vi "Vision ProcessingCheeto.vi"(4 "error in (no error)":errorcluster, 7 "Image Size Gear":T2=enum."160x120") -> ()   [LabVIEW 2016]
doc: "This VI runs in parallel to other tasks. It gets images from the camera, processes them for color or shape and use that information to affect robot behavior."
uses:
  Vision Support VIs/Camera Types.ctl
  <vilib>/Rock Robotics/WPI/Camera/WPI_CameraImageSize.ctl
  <vilib>/vision/Measure.llb/Edge Options.ctl
  <vilib>/vision/Measure.llb/Edge Polarity.ctl
  <vilib>/Rock Robotics/WPI/Camera/WPI_CameraWhite Balance Values.ctl
  <vilib>/Rock Robotics/WPI/Camera/WPI_CameraExposure Values.ctl
  <vilib>/Rock Robotics/WPI/Camera/WPI_CameraFrameRate.ctl
  <vilib>/Platform/TimedLoop/XDataNode/timing_clust.ctl
  <vilib>/Platform/TimedLoop/XDataNode/nitl_modes.ctl
  <vilib>/Platform/TimedLoop/XDataNode/wakeup.ctl
  Robot Global Data.vi
  <vilib>/platform/TimedLoop/XDataNode/XDataNode.xnode
  <vilib>/vision/NI_Vision_Development_Module.lvlib
  <vilib>/Platform/TimedLoop/XDataNode/XDNodeRunTimeDep.lvlib
panel:
  out "Distance (lateral) 2":dbl
  out "Distance (lateral) 1":dbl
  out "Gear Sorted Data":dbl[][](array[numeric])
  out "Original Image 3":T1(plugin-control)
  in  "error in (no error) 3":errorcluster
  in  "Image Size 2":T2=enum."320x240"
  in  "Image Size":T2=enum."320x240"
  in  "error in (no error) 2":errorcluster
  out "Original Image 2":T1(plugin-control)
  out "Gear Yaw Delta":dbl=-5.600000000000001
  in  "Boiler boresight":dbl=8.65
  in  "Edge Options Gear":T3={"Edge Polarity"=0, "Kernel Size"=3, "Width"=3, "Minimum Edge Strength"=15.0, "Interpolation Type"=enum."Bilinear Fixed", "Data Processing Method"=enum."Average"} {"Edge Polarity" items=["All Edges", "Rising Edges", "Falling Edges"]; "Minimum Edge Strength" format="%.2f"; "Width" step=2; "Kernel Size" step=2}
  in  "Gear boresight":dbl=24.9
  in  "Factor to Distance":dbl=12.0
  in  "Ball?":bool=TRUE
  in  "LED Color Ball":T5={"Hue"={190.47824477034428, 247.1686130718606}, "Sat"={57.67857142857144, 203.39285714285714}, "Val"={27.32142857142858, 255.0}} {"Hue" scale=0.0..255.0 scale format="%#_3g"}
  in  "Brightness":i32=30
  in  "Exposure (%)":dbl format="%#_13g"
  in  "Color Temp (K)":dbl=4000.0 format="%#_13g"
  in  "Edge Options":T3={"Edge Polarity"=0, "Kernel Size"=3, "Width"=3, "Minimum Edge Strength"=2.0, "Interpolation Type"=enum."Bilinear Fixed", "Data Processing Method"=enum."Average"} {"Edge Polarity" items=["All Edges", "Rising Edges", "Falling Edges"]; "Minimum Edge Strength" format="%.2f"; "Width" step=2; "Kernel Size" step=2}
  in  "Size Limit %":dbl=0.04 format="%#_13g"
  in  "Cal Turret":bool
  out "Calibration error 2":errorcluster={"status"=TRUE, "code"=-1074396074, "source"=""}
  out "Physical Paths":string[](array[string])=["-0_1_1_1_0", "-0_1_2_1_0"]
  out "Logical Paths":string[](array[string])=["video0", "video1"]
  out "Gear Valid":bool
  out "Boiler Yaw Delta":dbl=-8.499999999999998
  out "Boiler Valid":bool
  out "Boiler Distance":dbl=inf
  in  "Angle":enum16{"Horizontal", "Vertical", "Diagonal"}(ring)=enum."Vertical"
  in  "Gear?":bool
  in  "Image SizeTurr":T2=enum."160x120"
  in  "Score Cutoff Turret":dbl=70.0
  out "Gear Distance":dbl=inf
  in  "FOV":cluster{"X (degrees)":dbl, "Y (degrees)":dbl}={"X (degrees)"=34.3, "Y (degrees)"=61.0}
  in  "Height":T6={"Hc (GND to lense)"=12.5, "Ht (GND to CTR)"=0.0}
  in  "LED Color Target":T5={"Hue"={217.1650671807445, 7.296259223023774}, "Sat"={115.35714285714286, 255.0}, "Val"={21.25000000000001, 255.0}} {"Hue" scale=0.0..255.0 scale format="%#_3g"}
  in  "Camera Type":T7=enum."1013"
  in  "Score Cutoff %":dbl=50.0
  in  "Particles":dbl=5.0
  in  "Color Mode":u16(ring)=3 items=["RGB", "HSL", "HSV", "HSI"]
  in  "Use Calibration":bool
  out "Calibration error":errorcluster
  in  "Line Border":cluster{"Top":dbl, "Bottom":dbl}={"Top"=6.0, "Bottom"=1.0}
  in  "Display Original":bool=TRUE
  in  "Display Mask":bool=TRUE
  out "Mask":T1(plugin-control)
  out "Original Image":T1(plugin-control)
  out "loop ms":u32=200
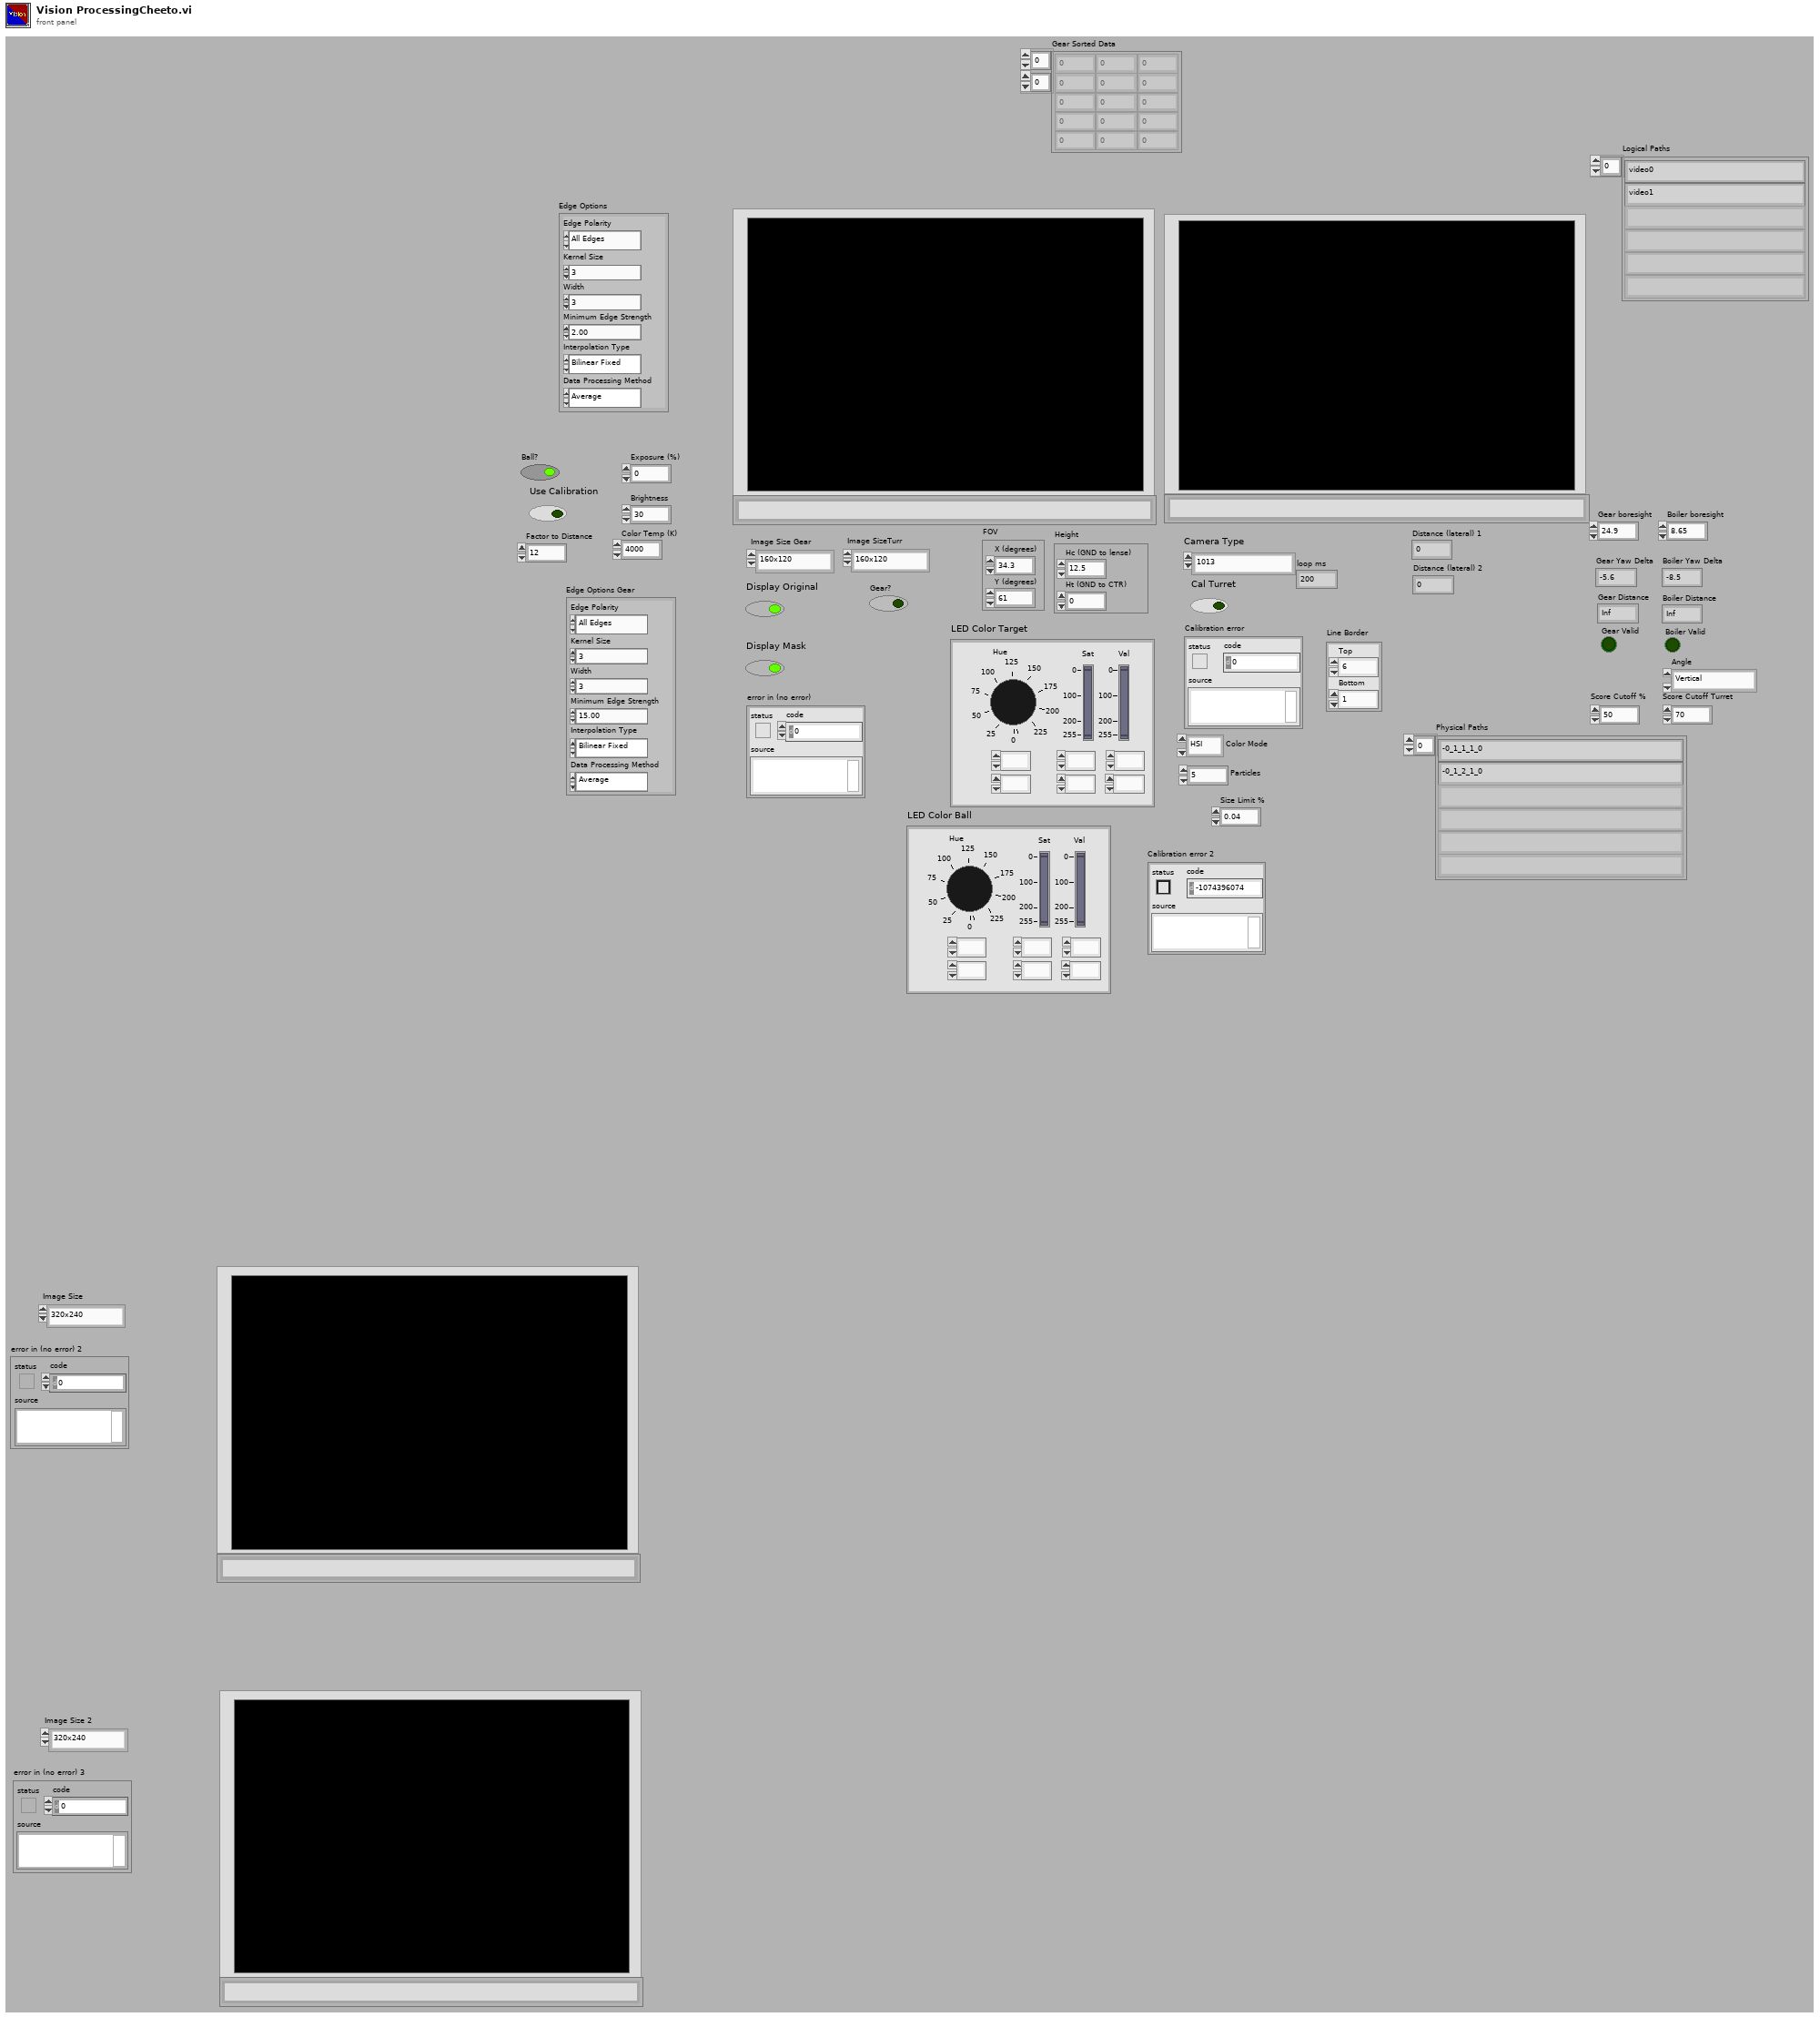
[diagram p1: front panel]
types:
  T1 = typedef "IMAQ Image.ctl" = refnum<image>
  T2 = typedef "WPI_CameraImageSize.ctl" = enum16{"640x480", "320x240", "160x120", "Custom"}
  T3 = typedef "Edge Options.ctl" = cluster{"Edge Polarity":T4, "Kernel Size":u32, "Width":u32, "Minimum Edge Strength":sgl, "Interpolation Type":enum32{"Zero Order", "Bilinear", "Quadratic", "Cubic", "Bilinear Fixed"}, "Data Processing Method":enum32{"Average", "Median"}}
  T4 = typedef "Edge Polarity.ctl" = u32
  T5 = cluster{"Hue":cluster{dbl, dbl}, "Sat":cluster{dbl, dbl}, "Val":cluster{dbl, dbl}}
  T6 = cluster{"Hc (GND to lense)":dbl, "Ht (GND to CTR)":dbl}
  T7 = typedef "Camera Types.ctl" = enum16{"206", "1011", "1013", "MS HD3000 square", "MS HD3000 640x480"}
  T8 = typedef "WPI_CameraFrameRate.ctl" = u32
  T9 = typedef "WPI_CameraExposure Values.ctl" = enum16{"Auto", "Flicker-free 50 Hz", "Flicker-free 60 Hz", "Hold current", "Custom"}
  T10 = typedef "WPI_CameraWhite Balance Values.ctl" = enum16{"Auto", "Fixed indoor", "Fixed outdoor 1", "Fixed outdoor 2", "Fixed fluorescent 1", "Fixed fluorescent 2", "Hold current", "Custom"}
  T11 = typedef "XDNodeRunTimeDep.lvlib/timing_clust.ctl" = cluster{"Expected End [f-1]":u64, "Actual End [f-1]":u64, "Finished Late? [f-1]":bool, "Expected End [i-1]":u64, "Actual End [i-1]":u64, "Finished Late? [i-1]":bool, "Expected Start [i]":u64, "Actual Start [i]":u64, "Expected Start [f]":u64, "Actual Start [f]":u64, "Source Name":string, "Structure Name":string, "Period":i64, "Deadline":i64, "Offset":i64, "Start":i64, "Priority":i32, "Timeout":i32, "Mode":T12, "Wakeup Reason":T13, "Error":errorcluster, "Source Type":string, "Secondary Source Type":string, "Global End Time":u64, "Global Start Time":u64, "Frame Duration":u64, "Iteration Duration":u64, "Assigned CPU":i32, "I/O Scan Engine Mode":u32}
  T12 = typedef "XDNodeRunTimeDep.lvlib/nitl_modes.ctl" = enum32{"No Change", "Process missed periods, maintain original phase", "Discard missed periods, maintain original phase", "Process missed periods, ignore original phase", "Discard missed periods, ignore original phase"}
  T13 = typedef "XDNodeRunTimeDep.lvlib/wakeup.ctl" = enum32{"Normal", "Aborted", "Asynchronous wakeup", "Timing source error", "Timed loop error", "Timeout"}
  T14 = typedef "Image Type" = u32
  T15 = typedef "WPI_CameraDevRef.ctl" = cluster{"Camera Address":string, "CameraStatus":errorcluster}
  T16 = typedef "Particle Parameters" = i32
  T17 = cluster{"Left":dbl, "Top":dbl, "Right":dbl, "Bottom":dbl}
  T18 = cluster{"Distance (ft)":dbl, "Score":dbl, "Normalized":cluster{"Center":cluster{dbl, dbl}, "Rectangle":cluster{"Numeric":dbl, "Numeric 2":dbl, "Numeric 3":dbl, "Numeric 5":dbl}}, "Pixels":cluster{"Center":cluster{dbl, dbl}, "Rectangle":cluster{"Numeric":dbl, "Numeric 2":dbl, "Numeric 3":dbl, "Numeric 5":dbl}}}
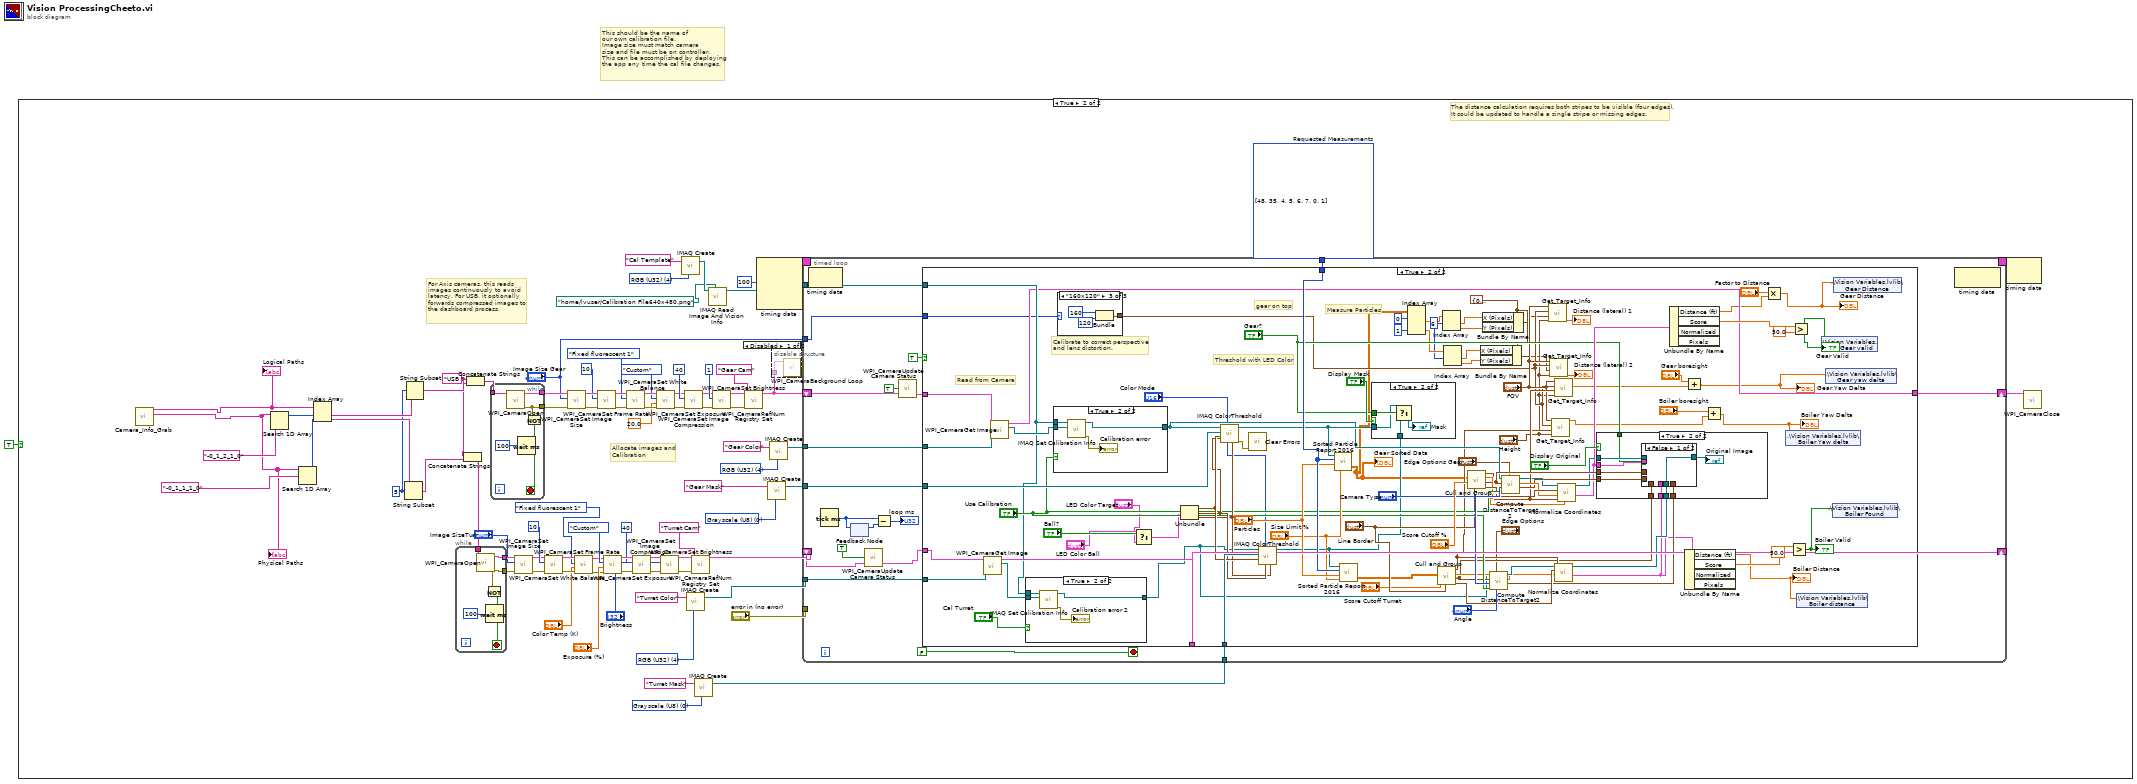
[diagram p0: block diagram]
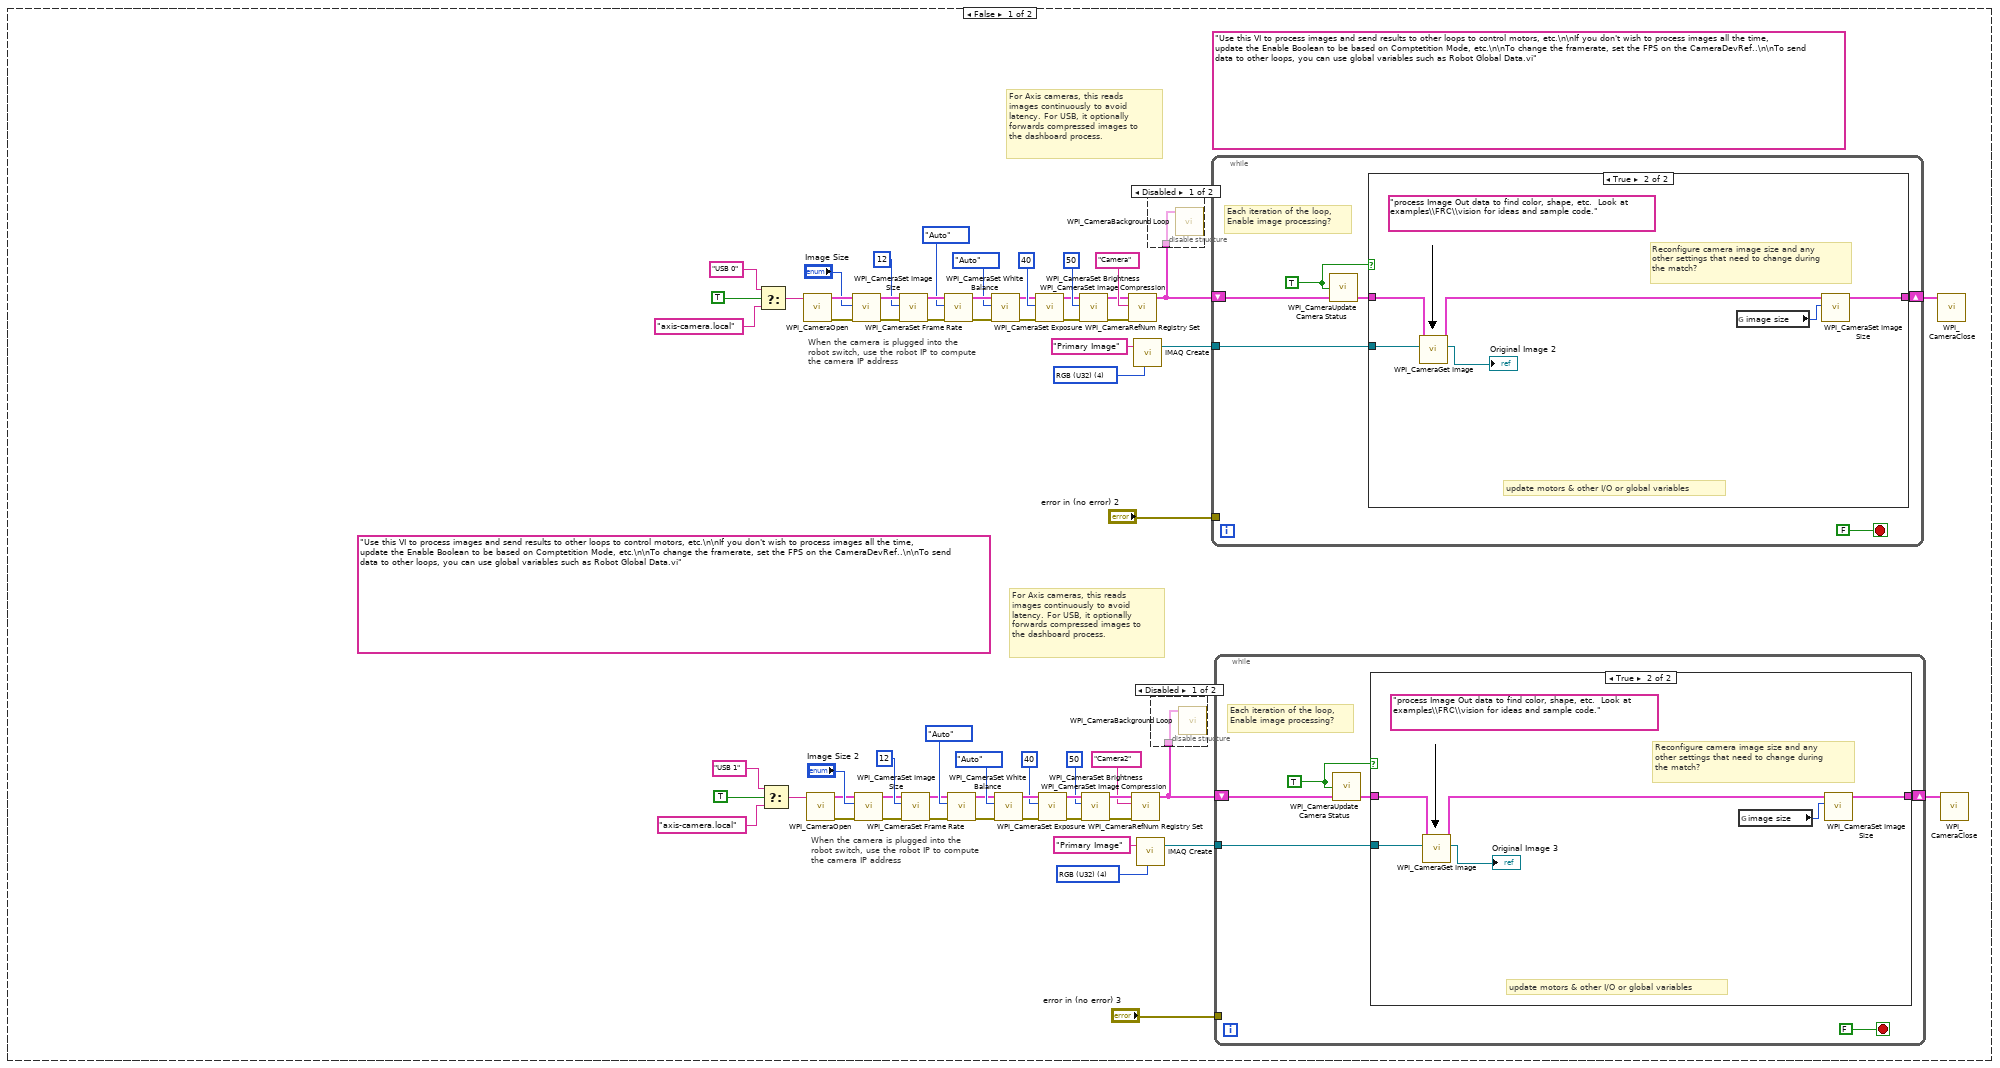
[diagram p2: hidden frame]
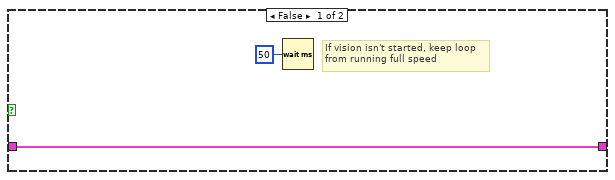
[diagram p4: hidden frame]
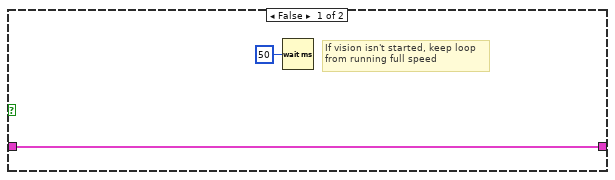
[diagram p6: hidden frame]
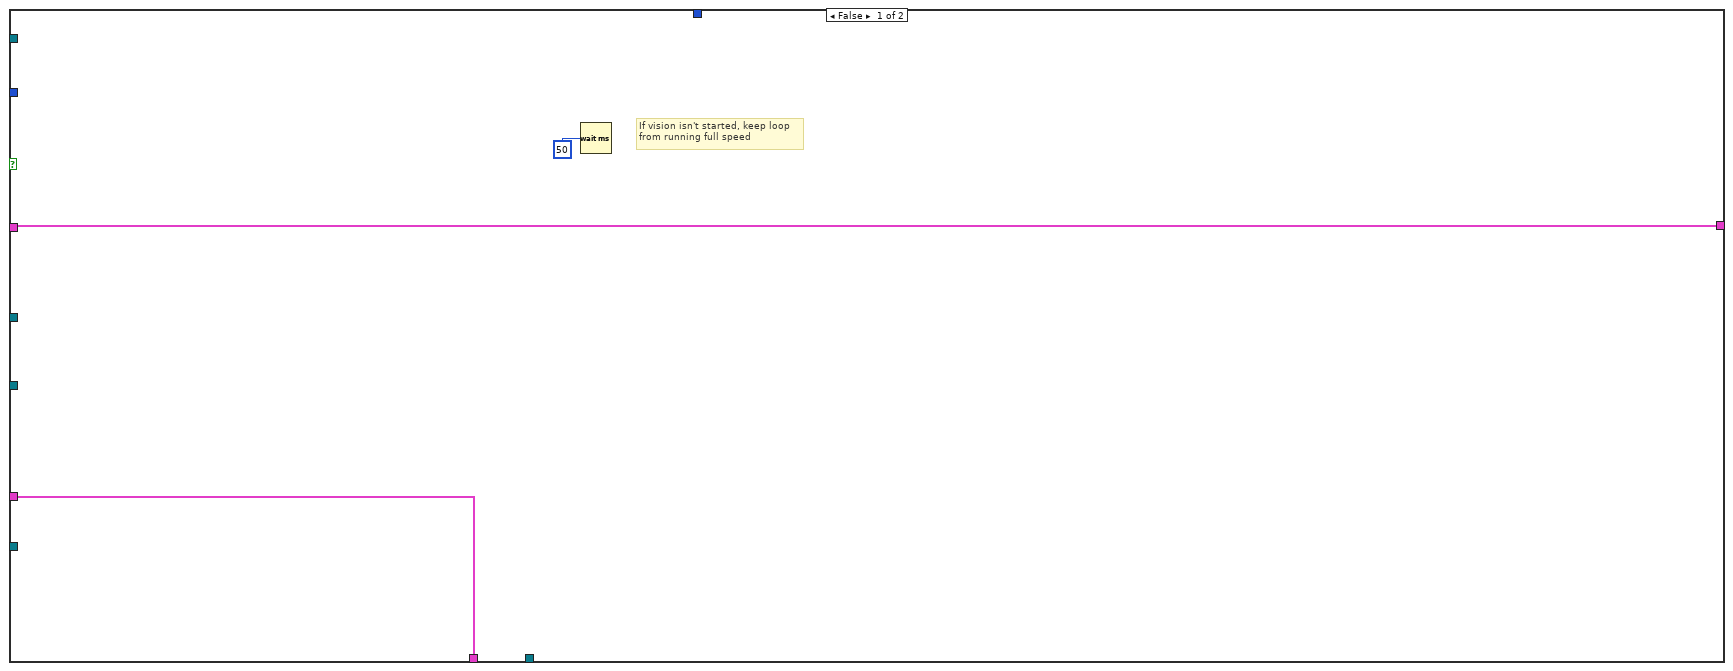
[diagram p7: hidden frame]
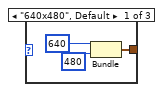
[diagram p8: hidden frame]
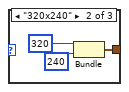
[diagram p9: hidden frame]
diagram:
  # "This should be the name of \nour own calibration file.\nImage size must match camera\nsize and file must be on controller.\nThis can be accomplished by deploying\nthe app any time the cal file changes."
  n1 = case shown="True" TRUE {
    frame False {
      (unwired) "Use this VI to process images and send results to other loops to control motors, etc.\n\nIf you don't wish to process images all the time, update the Enable Boolean to be based on Comptetition Mode, etc.\n\nTo change the framerate, set the FPS on the CameraDevRef..\n\nTo send data to other loops, you can use global variables such as Robot Global Data.vi"
      w2 = T14 4 items=["Grayscale (U8)", "Grayscale (I16)", "Grayscale (SGL)", "Complex (CSG)", "RGB (U32)", "HSL (U32)", "RGB (U64)"] ("Image Type")
      (unwired) "Use this VI to process images and send results to other loops to control motors, etc.\n\nIf you don't wish to process images all the time, update the Enable Boolean to be based on Comptetition Mode, etc.\n\nTo change the framerate, set the FPS on the CameraDevRef..\n\nTo send data to other loops, you can use global variables such as Robot Global Data.vi"
      w63 = T14 4 items=["Grayscale (U8)", "Grayscale (I16)", "Grayscale (SGL)", "Complex (CSG)", "RGB (U32)", "HSL (U32)", "RGB (U64)"] ("Image Type")
      # "When the camera is plugged into the\nrobot switch, use the robot IP to compute\nthe camera IP address"
      # "For Axis cameras, this reads\nimages continuously to avoid\nlatency. For USB, it optionally\nforwards compressed images to\nthe dashboard process."
      # "When the camera is plugged into the\nrobot switch, use the robot IP to compute\nthe camera IP address"
      # "For Axis cameras, this reads\nimages continuously to avoid\nlatency. For USB, it optionally\nforwards compressed images to\nthe dashboard process."
      n2 = Select(t="USB 0" ("format string"), s=TRUE ("dot notation? (F)"), f="axis-camera.local" ("format string")) -> (s? t:f=w34:string)
      n3 = Select(t="USB 1" ("format string"), s=TRUE ("dot notation? (F)"), f="axis-camera.local" ("format string")) -> (s? t:f=w31:string)
      n4 = call <vilib>:"WPI_CameraOpen.vi"("Camera Address"=w34) -> ("error out"=w51:errorcluster, "CameraDevRef"=w52:T15)  [unwired: 1 in, 8 out]
      n5 = call <vilib>:"WPI_CameraOpen.vi"("Camera Address"=w31) -> ("error out"=w14:errorcluster, "CameraDevRef"=w13:T15)  [unwired: 1 in, 8 out]
      n6 = call <vilib>:"WPI_CameraSet Image Size.vi"("error in (no error)"=w51, "Image Size"="Image Size", "CameraDevRef"=w52) -> ("error out"=w50:errorcluster, "CameraDevRef Out"=w53:T15)  [unwired: 1 in, 6 out]
      n7 = call <vilib>:"WPI_CameraSet Image Size.vi"("error in (no error)"=w14, "Image Size"="Image Size 2", "CameraDevRef"=w13) -> ("error out"=w15:errorcluster, "CameraDevRef Out"=w12:T15)  [unwired: 1 in, 6 out]
      n8 = call <vilib>:"WPI_CameraSet Frame Rate.vi"("error in (no error)"=w50, "Frame Rate (fps)"=T8 12, "CameraDevRef"=w53) -> ("error out"=w49:errorcluster, "CameraDevRef Out"=w55:T15)  [unwired: 7 out]
      n9 = call <vilib>:"WPI_CameraSet Frame Rate.vi"("error in (no error)"=w15, "Frame Rate (fps)"=T8 12, "CameraDevRef"=w12) -> ("error out"=w16:errorcluster, "CameraDevRef Out"=w10:T15)  [unwired: 7 out]
      n10 = call <vilib>:"WPI_CameraSet White Balance.vi"("error in (no error)"=w49, "White Balance"=WPI_CameraWhite_Balance_Values."Auto", "CameraDevRef"=w55) -> ("error out"=w48:errorcluster, "CameraDevRef Out"=w54:T15)  [unwired: 1 in, 6 out]
      n11 = call <vilib>:"WPI_CameraSet White Balance.vi"("error in (no error)"=w16, "White Balance"=WPI_CameraWhite_Balance_Values."Auto", "CameraDevRef"=w10) -> ("error out"=w17:errorcluster, "CameraDevRef Out"=w11:T15)  [unwired: 1 in, 6 out]
      n12 = call <vilib>:"WPI_CameraSet Exposure.vi"("error in (no error)"=w48, "Exposure"=WPI_CameraExposure_Values."Auto", "CameraDevRef"=w54) -> ("error out"=w47:errorcluster, "CameraDevRef Out"=w57:T15)  [unwired: 1 in, 6 out]
      n13 = call <vilib>:"WPI_CameraSet Exposure.vi"("error in (no error)"=w17, "Exposure"=WPI_CameraExposure_Values."Auto", "CameraDevRef"=w11) -> ("error out"=w18:errorcluster, "CameraDevRef Out"=w8:T15)  [unwired: 1 in, 6 out]
      n14 = call <vilib>:"WPI_CameraSet Image Compression.vi"("error in (no error)"=w47, "Compression"=40, "CameraDevRef"=w57) -> ("error out"=w46:errorcluster, "CameraDevRef Out"=w56:T15)  [unwired: 7 out]
      n15 = call <vilib>:"WPI_CameraSet Image Compression.vi"("error in (no error)"=w18, "Compression"=40, "CameraDevRef"=w8) -> ("error out"=w19:errorcluster, "CameraDevRef Out"=w9:T15)  [unwired: 7 out]
      n16 = call <vilib>:"WPI_CameraSet Brightness.vi"("error in (no error)"=w46, "Brightness"=50, "CameraDevRef"=w56) -> ("error out"=w44:errorcluster, "CameraDevRef Out"=w45:T15)  [unwired: 7 out]
      n17 = call <vilib>:"WPI_CameraSet Brightness.vi"("error in (no error)"=w19, "Brightness"=50, "CameraDevRef"=w9) -> ("error out"=w21:errorcluster, "CameraDevRef Out"=w20:T15)  [unwired: 7 out]
      n18 = call <vilib>:"WPI_CameraRefNum Registry Set.vi"("error in (no error)"=w44, "refnum name"="Camera", "CameraDevRef"=w45) -> ("CameraDevRef"=w40:T15)  [unwired: 1 in, 7 out]
      n19 = call <vilib>:"WPI_CameraRefNum Registry Set.vi"("error in (no error)"=w21, "refnum name"="Camera2", "CameraDevRef"=w20) -> ("CameraDevRef"=w25:T15)  [unwired: 1 in, 7 out]
      n20 = call "IMAQ Create"("Image Name"="Primary Image", "Image Type"=w63) -> ("New Image"=w61:T1)  [unwired: 2 in, 2 out]
      n21 = call "IMAQ Create"("Image Name"="Primary Image", "Image Type"=w2) -> ("New Image"=w4:T1)  [unwired: 2 in, 2 out]
      n22 = disable-structure shown="Disabled" {
        disable-tunnel: w40 -> [w79 _]
        frame Disabled {
          n23 = call <vilib>:"WPI_CameraBackground Loop.vi"("CameraDevRef"=w79) -> ()  [unwired: 11 in]
        }
        frame Enabled {
        }
      }
      n24 = disable-structure shown="Disabled" {
        disable-tunnel: w25 -> [w64 _]
        frame Disabled {
          n25 = call <vilib>:"WPI_CameraBackground Loop.vi"("CameraDevRef"=w64) -> ()  [unwired: 11 in]
        }
        frame Enabled {
        }
      }
      n26 = while {
        shift-right: [w84] -> w38
        shift-left: w40 -> [w82]
        tunnel: w61 -> [w83]
        tunnel: "error in (no error) 2" -> [_]
        stop <- FALSE stop-if-true
        w80 = TRUE
        # "Each iteration of the loop,\nEnable image processing?"
        n27 = call <vilib>:"WPI_CameraUpdate Camera Status.vi"("CameraDevRef In"=w82, "Enable Vision"=w80) -> ("CameraDevRef Out"=w81:T15)  [unwired: 3 in]
        n28 = case shown="True" w80 {
          tunnel: w83 -> [_ w92]
          tunnel: [w87 w93] -> w84
          tunnel: w81 -> [w87 w90]
          frame False {
            # "If vision isn't started, keep loop\nfrom running full speed"
            n29 = Wait (ms)(milliseconds to wait=u32 50) -> ()  [unwired: 1 out]
          }
          frame True {
            (unwired) "process Image Out data to find color, shape, etc.  Look at examples\\FRC\\vision for ideas and sample code."
            # "update motors & other I/O or global variables"
            # "Reconfigure camera image size and any\nother settings that need to change during\nthe match?"
            n30 = call <vilib>:"WPI_CameraGet Image.vi"("Image"=w92, "CameraDevRef"=w90) -> ("Image Out"=→"Original Image 2":T1, "CameraDevRef Out"=w89:T15)  [unwired: 1 in, 7 out]
            n31 = global read "Robot Global Data.vi" "image size"() -> (w91:T2)
            n32 = call <vilib>:"WPI_CameraSet Image Size.vi"("Image Size"=w91, "CameraDevRef"=w89) -> ("CameraDevRef Out"=w93:T15)  [unwired: 2 in, 7 out]
          }
        }
      }
      n33 = while {
        shift-right: [w69] -> w27
        shift-left: w25 -> [w67]
        tunnel: w4 -> [w68]
        tunnel: "error in (no error) 3" -> [_]
        stop <- FALSE stop-if-true
        w65 = TRUE
        # "Each iteration of the loop,\nEnable image processing?"
        n34 = call <vilib>:"WPI_CameraUpdate Camera Status.vi"("CameraDevRef In"=w67, "Enable Vision"=w65) -> ("CameraDevRef Out"=w66:T15)  [unwired: 3 in]
        n35 = case shown="True" w65 {
          tunnel: w68 -> [_ w77]
          tunnel: [w72 w78] -> w69
          tunnel: w66 -> [w72 w75]
          frame False {
            # "If vision isn't started, keep loop\nfrom running full speed"
            n36 = Wait (ms)(milliseconds to wait=u32 50) -> ()  [unwired: 1 out]
          }
          frame True {
            (unwired) "process Image Out data to find color, shape, etc.  Look at examples\\FRC\\vision for ideas and sample code."
            # "update motors & other I/O or global variables"
            # "Reconfigure camera image size and any\nother settings that need to change during\nthe match?"
            n37 = call <vilib>:"WPI_CameraGet Image.vi"("Image"=w77, "CameraDevRef"=w75) -> ("Image Out"=→"Original Image 3":T1, "CameraDevRef Out"=w74:T15)  [unwired: 1 in, 7 out]
            n38 = global read "Robot Global Data.vi" "image size"() -> (w76:T2)
            n39 = call <vilib>:"WPI_CameraSet Image Size.vi"("Image Size"=w76, "CameraDevRef"=w74) -> ("CameraDevRef Out"=w78:T15)  [unwired: 2 in, 7 out]
          }
        }
      }
      n40 = call <vilib>:"WPI_CameraClose.vi"("CameraDevRef"=w38) -> ()  [unwired: 1 in, 10 out]
      n41 = call <vilib>:"WPI_CameraClose.vi"("CameraDevRef"=w27) -> ()  [unwired: 1 in, 10 out]
    }
    frame True {
      w108 = "USB " ("string")
      w110 = 5 ("offset (0)")
      w118 = T14 0 items=["Grayscale (U8)", "Grayscale (I16)", "Grayscale (SGL)", "Complex (CSG)", "RGB (U32)", "HSL (U32)", "RGB (U64)", "Grayscale (U16)"] ("Image Type")
      w120 = T14 4 items=["Grayscale (U8)", "Grayscale (I16)", "Grayscale (SGL)", "Complex (CSG)", "RGB (U32)", "HSL (U32)", "RGB (U64)", "Grayscale (U16)"] ("Image Type")
      w168 = T14 4 items=["Grayscale (U8)", "Grayscale (I16)", "Grayscale (SGL)", "Complex (CSG)", "RGB (U32)", "HSL (U32)", "RGB (U64)", "Grayscale (U16)"] ("Image Type")
      w173 = T14 0 items=["Grayscale (U8)", "Grayscale (I16)", "Grayscale (SGL)", "Complex (CSG)", "RGB (U32)", "HSL (U32)", "RGB (U64)", "Grayscale (U16)"] ("Image Type")
      w174 = T14 4 items=["Grayscale (U8)", "Grayscale (I16)", "Grayscale (SGL)", "Complex (CSG)", "RGB (U32)", "HSL (U32)", "RGB (U64)", "Grayscale (U16)"] ("Image Type")
      w170 = T16[] [48, 35, 4, 5, 6, 7, 0, 1] items=["Center of Mass X", "Center of Mass Y", "First Pixel X", "First Pixel Y", "Bounding Rect Left", "Bounding Rect Top", "Bounding Rect Right", "Bounding Rect Bottom", "Max Feret Diameter Start X", "Max Feret Diameter Start Y", "Max Feret Diameter End X", "Max Feret Diameter End Y", "Max Horiz. Segment Length Left", "Max Horiz. Segment Length Right", "Max Horiz. Segment Length Row", "-", "Bounding Rect Width", "Bounding Rect Height", "Bounding Rect Diagonal", "Perimeter", "Convex Hull Perimeter", "Holes' Perimeter", "Max Feret Diameter", "Equivalent Ellipse Major Axis", "Equivalent Ellipse Minor Axis", "Equivalent Ellipse Minor Axis (Feret)", "Equivalent Rect Long Side", "Equivalent Rect Short Side", "Equivalent Rect Diagonal", "Equivalent Rect Short Side (Feret)", "Average Horiz. Segment Length", "Average Vert. Segment Length", "Hydraulic Radius", "Waddel Disk Diameter", "-", "Area", "Holes' Area", "Particle & Holes' Area", "Convex Hull Area", "Image Area", "-", "Number of Holes", "Number of Horiz. Segments", "Number of Vert. Segments", "-", "Orientation", "Max Feret Diameter Orientation", "-", "% Area/Image Area", "% Area/(Particle & Holes' Area)", "Ratio of Equivalent Ellipse Axes", "Ratio of Equivalent Rect Sides", "-", "Elongation Factor", "Compactness Factor", "Heywood Circularity Factor", "Type Factor", "-", "Sum X", "Sum Y", "Sum XX", "Sum XY", "Sum YY", "Sum XXX", "Sum XXY", "Sum XYY", "Sum YYY", "-", "Moment of Inertia XX", "Moment of Inertia XY", "Moment of Inertia YY", "Moment of Inertia XXX", "Moment of Inertia XXY", "Moment of Inertia XYY", "Moment of Inertia YYY", "Norm. Moment of Inertia XX", "Norm. Moment of Inertia XY", "Norm. Moment of Inertia YY", "Norm. Moment of Inertia XXX", "Norm. Moment of Inertia XXY", "Norm. Moment of Inertia XYY", "Norm. Moment of Inertia YYY", "Hu Moment 1", "Hu Moment 2", "Hu Moment 3", "Hu Moment 4", "Hu Moment 5", "Hu Moment 6", "Hu Moment 7"]  # Requested Measurements
      # "For Axis cameras, this reads\nimages continuously to avoid\nlatency. For USB, it optionally\nforwards compressed images to\nthe dashboard process."
      # "Allocate images and\nCalibration"
      # "The distance calculation requires both stripes to be visible (four edges).\nIt could be updated to handle a single stripe or missing edges."
      n42 = call <userlib>:"Camera_Info_Grab.vi"() -> ("Physical Paths"=w102:string[], "Logical Paths"=w103:string[])  [unwired: 10 in]
      "Logical Paths" <- w103
      "Physical Paths" <- w102
      n43 = Search 1D Array(1D array=w102, element="-0_1_2_1_0") -> (index of element=w114:i32)  [unwired: 1 in]
      n44 = Search 1D Array(1D array=w102, element="-0_1_1_1_0") -> (index of element=w113:i32)  [unwired: 1 in]
      n45 = Index Array(array=w103, index #1=w114, index #2=w113) -> (element #1=w112:string, element #2=w111:string)
      n46 = String Subset(string=w111, offset (0)=w110) -> (substring=w107:string)  [unwired: 1 in]
      n47 = String Subset(string=w112, offset (0)=w110) -> (substring=w109:string)  [unwired: 1 in]
      n48 = Concatenate Strings(w108, w107) -> (w106:string)
      n49 = while {
        tunnel: [w341] -> w133
        tunnel: [w344] -> w132
        tunnel: w106 -> [w343]
        stop <- w340 stop-if-true
        n50 = call <vilib>:"WPI_CameraOpen.vi"("Camera Address"=w343) -> ("error out"=w341:errorcluster, "CameraDevRef"=w344:T15)  [unwired: 1 in, 8 out]
        n51 = Not(x=w341) -> (.not. x?=w340:bool)
        n52 = Wait (ms)(milliseconds to wait=u32 100) -> ()  [unwired: 1 out]
      }
      n53 = Concatenate Strings(w108, w109) -> (w105:string)
      n54 = while {
        tunnel: [w339] -> w155
        tunnel: [w336] -> w154
        tunnel: w105 -> [w338]
        stop <- w335 stop-if-true
        n55 = call <vilib>:"WPI_CameraOpen.vi"("Camera Address"=w338) -> ("error out"=w336:errorcluster, "CameraDevRef"=w339:T15)  [unwired: 1 in, 8 out]
        n56 = Wait (ms)(milliseconds to wait=u32 100) -> ()  [unwired: 1 out]
        n57 = Not(x=w336) -> (.not. x?=w335:bool)
      }
      n58 = call <vilib>:"WPI_CameraSet Image Size.vi"("error in (no error)"=w133, "Image Size"="Image SizeTurr", "CameraDevRef"=w132) -> ("error out"=w134:errorcluster, "CameraDevRef Out"=w131:T15)  [unwired: 1 in, 6 out]
      n59 = call <vilib>:"WPI_CameraSet Frame Rate.vi"("error in (no error)"=w134, "Frame Rate (fps)"=T8 10, "CameraDevRef"=w131) -> ("error out"=w98:errorcluster, "CameraDevRef Out"=w100:T15)  [unwired: 7 out]
      n60 = call <vilib>:"WPI_CameraSet Image Size.vi"("error in (no error)"=w154, "Image Size"="Image Size Gear", "CameraDevRef"=w155) -> ("error out"=w153:errorcluster, "CameraDevRef Out"=w156:T15)  [unwired: 1 in, 6 out]
      n61 = call <vilib>:"WPI_CameraSet White Balance.vi"("error in (no error)"=w98, "Color Temp (K)"="Color Temp (K)", "White Balance"=WPI_CameraWhite_Balance_Values."Fixed fluorescent 1", "CameraDevRef"=w100) -> ("error out"=w97:errorcluster, "CameraDevRef Out"=w99:T15)  [unwired: 6 in]
      n62 = call <vilib>:"WPI_CameraSet Frame Rate.vi"("error in (no error)"=w153, "Frame Rate (fps)"=T8 10, "CameraDevRef"=w156) -> ("error out"=w152:errorcluster, "CameraDevRef Out"=w158:T15)  [unwired: 7 out]
      n63 = call <vilib>:"WPI_CameraSet Exposure.vi"("error in (no error)"=w97, "Exposure (%)"="Exposure (%)", "Exposure"=WPI_CameraExposure_Values."Custom", "CameraDevRef"=w99) -> ("error out"=w135:errorcluster, "CameraDevRef Out"=w129:T15)  [unwired: 6 out]
      n64 = call <vilib>:"WPI_CameraSet White Balance.vi"("error in (no error)"=w152, "White Balance"=WPI_CameraWhite_Balance_Values."Fixed fluorescent 1", "CameraDevRef"=w158) -> ("error out"=w151:errorcluster, "CameraDevRef Out"=w157:T15)  [unwired: 1 in, 6 out]
      n65 = call <vilib>:"WPI_CameraSet Image Compression.vi"("error in (no error)"=w135, "Compression"=40, "CameraDevRef"=w129) -> ("error out"=w136:errorcluster, "CameraDevRef Out"=w130:T15)  [unwired: 7 out]
      n66 = call <vilib>:"WPI_CameraSet Exposure.vi"("error in (no error)"=w151, "Exposure (%)"=20.0, "Exposure"=WPI_CameraExposure_Values."Custom", "CameraDevRef"=w157) -> ("error out"=w150:errorcluster, "CameraDevRef Out"=w160:T15)  [unwired: 6 out]
      n67 = call <vilib>:"WPI_CameraSet Brightness.vi"("error in (no error)"=w136, "Brightness"="Brightness", "CameraDevRef"=w130) -> ("error out"=w137:errorcluster, "CameraDevRef Out"=w124:T15)  [unwired: 7 out]
      n68 = call "IMAQ Create"("Image Name"="Cal Template", "Image Type"=w168) -> ("New Image"=w166:T1)  [unwired: 2 in, 2 out]
      n69 = call <vilib>:"WPI_CameraSet Image Compression.vi"("error in (no error)"=w150, "Compression"=40, "CameraDevRef"=w160) -> ("error out"=w149:errorcluster, "CameraDevRef Out"=w159:T15)  [unwired: 7 out]
      n70 = call "IMAQ Create"("Image Name"="Turret Color", "Image Type"=w120) -> ("New Image"=w119:T1)  [unwired: 2 in, 2 out]
      n71 = call <vilib>:"WPI_CameraRefNum Registry Set.vi"("error in (no error)"=w137, "refnum name"="Turret Cam", "CameraDevRef"=w124) -> ("CameraDevRef"=w122:T15)  [unwired: 1 in, 7 out]
      n72 = call "IMAQ Create"("Image Name"="Turret Mask", "Image Type"=w118) -> ("New Image"=w116:T1)  [unwired: 2 in, 2 out]
      n73 = call "IMAQ Read Image And Vision Info"("File Path"=path "/home/lvuser/Calibration File640x480.png" ("Folder Location"), "Image"=w166) -> ("Image Out"=w165:T1)  [unwired: 7 in, 2 out]
      n74 = call <vilib>:"WPI_CameraSet Brightness.vi"("error in (no error)"=w149, "Brightness"=1, "CameraDevRef"=w159) -> ("error out"=w148:errorcluster, "CameraDevRef Out"=w164:T15)  [unwired: 7 out]
      n75 = call <vilib>:"WPI_CameraRefNum Registry Set.vi"("error in (no error)"=w148, "refnum name"="Gear Cam", "CameraDevRef"=w164) -> ("CameraDevRef"=w144:T15)  [unwired: 1 in, 7 out]
      n76 = node-c288(i64 100 ("Period")) -> (w177:T11)  [unwired: 3 in]
      n77 = call "IMAQ Create"("Image Name"="Gear Mask", "Image Type"=w173) -> ("New Image"=w171:T1)  [unwired: 2 in, 2 out]
      n78 = call "IMAQ Create"("Image Name"="Gear Color", "Image Type"=w174) -> ("New Image"=w169:T1)  [unwired: 2 in, 2 out]
      n79 = disable-structure shown="Disabled" {
        disable-tunnel: w144 -> [w345 _]
        frame Disabled {
          n80 = call <vilib>:"WPI_CameraBackground Loop.vi"("CameraDevRef"=w345) -> ()  [unwired: 11 in]
        }
        frame Enabled {
        }
      }
      n81 = timed-loop {
        tunnel: w169 -> [w193]
        tunnel: w171 -> [w196]
        tunnel: w170 -> [w195]
        tunnel: w165 -> [w194]
        shift-right: [w192] -> w143
        shift-left: w144 -> [w191]
        tunnel: "error in (no error)" -> [_]
        tunnel: "Image Size Gear" -> [w178]
        shift-right: [w186] -> _
        shift-left: w122 -> [w181]
        tunnel: w119 -> [w185]
        tunnel: w116 -> [w184]
        timing: w177 -> [_]
        timing-out: [_] -> w176
        stop <- FALSE ("Boolean") stop-if-true
        n82 = node-c288() -> ()  [unwired: 1 in, 1 out]
        n83 = Tick Count (ms)() -> (millisecond timer value=w188:u32)
        n84 = feedback-in #1(w188) -> ()
        n85 = feedback #1() -> (w189:u32)  [unwired: 1 in]
        n86 = call <vilib>:"WPI_CameraUpdate Camera Status.vi"("CameraDevRef In"=w181, "Enable Vision"=TRUE) -> ("CameraDevRef Out"=w179:T15)  [unwired: 3 in]
        n87 = Subtract(x=w188, y=w189) -> (x-y=→"loop ms":u32)
        n88 = call <vilib>:"WPI_CameraUpdate Camera Status.vi"("CameraDevRef In"=w191, "Enable Vision"=TRUE) -> ("CameraDevRef Out"=w190:T15)  [unwired: 3 in]
        n89 = case shown="True" TRUE {
          tunnel: w196 -> [_ w295]
          tunnel: w195 -> [_ w284]
          tunnel: w194 -> [_ w245]
          tunnel: w190 -> [w202 w294]
          tunnel: w193 -> [_ w289]
          tunnel: [w202 w240] -> w192
          tunnel: w179 -> [w200 w292]
          tunnel: [w200 w291] -> w186
          tunnel: w185 -> [_ w290]
          tunnel: w184 -> [_ w288]
          tunnel: w178 -> [_ w220]
          frame False {
            # "If vision isn't started, keep loop\nfrom running full speed"
            n90 = Wait (ms)(milliseconds to wait=u32 50) -> ()  [unwired: 1 out]
          }
          frame True {
            w209 = 6 ("index")
            w213 = cluster{"X (Pixels)":dbl, "Y (Pixels)":dbl} {"X (Pixels)"=0.0, "Y (Pixels)"=0.0} ("Target Location")
            # "gear on top"
            # "Read from Camera"
            # "Calibrate to correct perspective\nand lens distortion."
            # "Measure Particles"
            # "Threshold with LED Color"
            n91 = call <vilib>:"WPI_CameraGet Image.vi"("Image"=w290, "CameraDevRef"=w292) -> ("Image Out"=w244:T1, "CameraDevRef Out"=w291:T15)  [unwired: 7 in, 1 out]
            n92 = call <vilib>:"WPI_CameraGet Image.vi"("Image"=w289, "CameraDevRef"=w294) -> ("Image Out"=w255:T1, "CameraDevRef Out"=w240:T15)  [unwired: 7 in, 1 out]
            n93 = case shown="True" "Cal Turret" {
              tunnel: [w305 w309] -> w243
              tunnel: w244 -> [w305 w308]
              tunnel: w245 -> [_ w307]
              frame False {
              }
              frame True {
                n94 = call "IMAQ Set Calibration Info"("Image Dst"=w308, "Image Src"=w307) -> ("error out"=→"Calibration error 2":errorcluster, "Calibrated Image"=w309:T1)  [unwired: 8 in]
              }
            }
            n95 = case shown="True" "Use Calibration" {
              tunnel: [w326 w330] -> w258
              tunnel: w255 -> [w326 w329]
              tunnel: w245 -> [_ w328]
              frame False {
              }
              frame True {
                n96 = call "IMAQ Set Calibration Info"("Image Dst"=w329, "Image Src"=w328) -> ("error out"=→"Calibration error":errorcluster, "Calibrated Image"=w330:T1)  [unwired: 8 in]
              }
            }
            n97 = case shown="\"160x120\"" w220 {
              tunnel: [w296 w299 w302] -> w219
              frame "640x480", Default {
                n98 = Bundle(640, 480) -> (w296:cluster{i32, i32})  [unwired: 1 in]
              }
              frame "320x240" {
                n99 = Bundle(320, 240) -> (w299:cluster{i32, i32})  [unwired: 1 in]
              }
              frame "160x120" {
                n100 = Bundle(160, 120) -> (w302:cluster{i32, i32})  [unwired: 1 in]
              }
            }
            n101 = Select(t="LED Color Ball", s="Ball?", f="LED Color Target") -> (s? t:f=w236:T5)
            n102 = Unbundle(w236) -> ("Hue"=w287:cluster{dbl, dbl}, "Sat"=w286:cluster{dbl, dbl}, "Val"=w285:cluster{dbl, dbl})
            n103 = call "IMAQ ColorThreshold"("Blue or Luma or Val or Inten Range"=w285, "Green or Sat Range"=w286, "Color Mode"="Color Mode", "Red or Hue Range"=w287, "Image Dst"=w295, "Image Src"=w258) -> ("error out"=w269:errorcluster, "Image Dst Out"=w268:T1)  [unwired: 4 in]
            n104 = call <vilib>:"Clear Errors.vi"("error in (no error)"=w269) -> ()  [unwired: 5 in, 2 out]
            n105 = call "IMAQ ColorThreshold"("Blue or Luma or Val or Inten Range"=w285, "Green or Sat Range"=w286, "Color Mode"="Color Mode", "Red or Hue Range"=w287, "Image Dst"=w288, "Image Src"=w243) -> ("Image Dst Out"=w251:T1)  [unwired: 4 in, 1 out]
            n106 = call "Sorted Particle Report 2016.vi"("Min Area Size %"="Size Limit %", "Particle Count Limit"="Particles", "Pixel Measurements"=w284, "Image in"=w268) -> ("Sorted Data"=w217:dbl[][])  [unwired: 1 out]
            "Gear Sorted Data" <- w217
            n107 = call "Sorted Particle Report 2016.vi"("Min Area Size %"="Size Limit %", "Particle Count Limit"="Particles", "Pixel Measurements"=w284, "Image in"=w251) -> ("Sorted Data"=w277:dbl[][])  [unwired: 1 out]
            n108 = case shown="True" "Display Mask" {
              tunnel: w268 -> [_ w323]
              tunnel: "Gear?" -> [_ w325]
              tunnel: w251 -> [_ w322]
              frame False {
              }
              frame True {
                n109 = Select(t=w323, s=w325, f=w322) -> (s? t:f=→"Mask":T1)
              }
            }
            n110 = Index Array(array=w217, index (row) #1=0 ("index (row)"), index (row) #2=1 ("index (row)")) -> (element #1=w214:dbl[], element #2=w212:dbl[])  [unwired: 2 in]
            n111 = call "Cull and Group.vi"("Line Border"="Line Border", "Score Cutoff"="Score Cutoff Turret", "Sorted Data"=w277) -> ("Rect"=w274:T17, "Line"=w249:T17, "Score"=w273:dbl, "Center"=w250:cluster{"X":dbl, "Y":dbl})  [unwired: 5 in]
            n112 = Index Array(array=w214, index #1=w209) -> (element #1=w211:dbl, element #2=w210:dbl)  [unwired: 1 in]
            n113 = Index Array(array=w212, index #1=w209) -> (element #1=w208:dbl, element #2=w207:dbl)  [unwired: 1 in]
            n114 = call "Cull and Group.vi"("Line Border"="Line Border", "Score Cutoff"="Score Cutoff %", "Sorted Data"=w217) -> ("Rect"=w267:T17, "Line"=w264:T17, "Score"=w265:dbl, "Center"=w257:cluster{"X":dbl, "Y":dbl})  [unwired: 5 in]
            n115 = Bundle By Name(cluster=w213, "X (Pixels)"=w208, "Y (Pixels)"=w207) -> (w205:cluster{"X (Pixels)":dbl, "Y (Pixels)":dbl})
            n116 = Bundle By Name(cluster=w213, "X (Pixels)"=w211, "Y (Pixels)"=w210) -> (w206:cluster{"X (Pixels)":dbl, "Y (Pixels)":dbl})
            n117 = call "Compute DistanceToTarget2.vi"("Angle"="Angle", "Edge Options"="Edge Options", "Calibrated"="Use Calibration", "Camera Type"="Camera Type", "Line"=w249, "Image Src"=w243) -> ("Edges"=w248:cluster{"X":sgl, "Y":sgl}[], "Distance (ft)"=w272:dbl, "Image Dst Out"=w275:T1)  [unwired: 3 in]
            n118 = call "Compute DistanceToTarget2.vi"("Edge Options"="Edge Options Gear", "Calibrated"="Use Calibration", "Camera Type"="Camera Type", "Line"=w264, "Image Src"=w258) -> ("Edges"=w263:cluster{"X":sgl, "Y":sgl}[], "Distance (ft)"=w266:dbl, "Image Dst Out"=w256:T1)  [unwired: 4 in]
            n119 = call "Get_Target_Info.vi"("Height"="Height", "Target Location"=w206, "Resolution"=w219, "FOV"="FOV") -> ("Distance (lateral)"=→"Distance (lateral) 1":dbl)  [unwired: 4 in, 3 out]
            n120 = call "Get_Target_Info.vi"("Height"="Height", "Target Location"=w205, "Resolution"=w219, "FOV"="FOV") -> ("Distance (lateral)"=→"Distance (lateral) 2":dbl)  [unwired: 4 in, 3 out]
            n121 = call "Get_Target_Info.vi"("Height"="Height", "Target Location"=w250, "Resolution"=w219, "FOV"="FOV") -> ("Yaw Delta"=w225:dbl)  [unwired: 4 in, 3 out]
            n122 = call "Get_Target_Info.vi"("Height"="Height", "Target Location"=w257, "Resolution"=w219, "FOV"="FOV") -> ("Elevation Delta"=w230:dbl)  [unwired: 4 in, 3 out]
            n123 = call "Normalize Coordinates.vi"("Score"=w273, "Center"=w250, "Distance"=w272, "Bounding box"=w274, "Image in"=w275) -> ("Results"=w222:T18, "Image out"=w247:T1)  [unwired: 5 in]
            n124 = call "Normalize Coordinates.vi"("Score"=w265, "Center"=w257, "Distance"=w266, "Bounding box"=w267, "Image in"=w256) -> ("Results"=w260:T18, "Image out"=w259:T1)  [unwired: 5 in]
            n125 = case shown="True" "Display Original" {
              tunnel: w259 -> [_ w318]
              tunnel: w260 -> [_ w317]
              tunnel: w264 -> [_ w316]
              tunnel: w263 -> [_ w315]
              tunnel: "Gear?" -> [_ w314]
              tunnel: w249 -> [_ w313]
              tunnel: w248 -> [_ w312]
              tunnel: w247 -> [_ w311]
              tunnel: w222 -> [_ w310]
              frame False {
              }
              frame True {
                n126 = case shown="False" w314 {
                  tunnel: [w320 w321] -> w319
                  tunnel: w318 -> [_ w321]
                  tunnel: w317 -> [_ _]
                  tunnel: w316 -> [_ _]
                  tunnel: w315 -> [_ _]
                  tunnel: w313 -> [_ _]
                  tunnel: w312 -> [_ _]
                  tunnel: w311 -> [w320 _]
                  tunnel: w310 -> [_ _]
                  frame False {
                  }
                  frame True {
                  }
                }
                "Original Image" <- w319
              }
            }
            n127 = Unbundle By Name(w260) -> ("Distance (ft)"=w234:dbl, "Score"=w254:dbl)  [unwired: 2 out]
            n128 = Unbundle By Name(w222) -> ("Distance (ft)"=w223:dbl, "Score"=w271:dbl)  [unwired: 2 out]
            "Boiler Distance" <- w223
            n129 = Add(x="Gear boresight", y=w230) -> (x+y=w233:dbl)
            "Gear Yaw Delta" <- w233
            n130 = Add(x="Boiler boresight", y=w225) -> (x+y=w224:dbl)
            "Boiler Yaw Delta" <- w224
            n131 = Multiply(x="Factor to Distance", y=w234) -> (x*y=w227:dbl)
            "Gear Distance" <- w227
            n132 = shared-variable ".\\Vision Variables.lvlib\\Boiler Yaw delta"(w224) -> ()  [unwired: 1 in, 1 out]
            n133 = Greater?(x=w271, y=50.0) -> (0:w228:bool)
            "Boiler Valid" <- w228
            n134 = Greater?(x=w254, y=50.0) -> (0:w229:bool)
            "Gear Valid" <- w229
            n135 = shared-variable ".\\Vision Variables.lvlib\\Boiler distance"(w223) -> ()  [unwired: 1 in, 1 out]
            n136 = shared-variable ".\\Vision Variables.lvlib\\Gear valid"(w229) -> ()  [unwired: 1 in, 1 out]
            n137 = shared-variable ".\\Vision Variables.lvlib\\Gear yaw delta"(w233) -> ()  [unwired: 1 in, 1 out]
            n138 = shared-variable ".\\Vision Variables.lvlib\\Boiler Found"(w228) -> ()  [unwired: 1 in, 1 out]
            n139 = shared-variable ".\\Vision Variables.lvlib\\Gear Distance"(w227) -> ()  [unwired: 1 in, 1 out]
          }
        }
        n140 = node-c288() -> ()  [unwired: 1 in, 1 out]
      }
      n141 = node-c288(w176) -> ()  [unwired: 1 out]
      n142 = call <vilib>:"WPI_CameraClose.vi"("CameraDevRef"=w143) -> ()  [unwired: 1 in, 10 out]
    }
  }
